vi "G2CPU GEMM And Operations Float.vi"(10 "Backend":T1 items=["Default Backend"=0, "CPU Backend"=1, "CUDA Backend"=2, "OPENCL Backend"=4, "Intel OneAPI"=8], 11 "dimension size":i32=16384) -> (3 "G2CPU Time":dbl)   [LabVIEW 2020]
uses:
  <vilib>/Natan Biesmans/G2CPU GPU and CPU HPC Toolkit/ArrayFire Driver/TypeDefs/backend.ctl
  ef11b89c-ff92-4b7a-88d6-625fca8c0d7c.vi
  c2200195-6f6b-46fb-afe8-d4cd0bcb91cf.vi
  fbbaf97c-3b5e-4b4c-bc14-40c3526c788b.vi
  ef11b89c-ff92-4b7a-88d6-625fca8c0d7c.vi/caaf1833-0905-411b-a9ed-2cc30d41907c.vi
  <vilib>/Natan Biesmans/G2CPU GPU and CPU HPC Toolkit/G2CPU Libraries/Arrays/SubVI/Array Sizes to Dim Cluster.vi
  c2200195-6f6b-46fb-afe8-d4cd0bcb91cf.vi/caaf1833-0905-411b-a9ed-2cc30d41907c.vi
  fbbaf97c-3b5e-4b4c-bc14-40c3526c788b.vi/caaf1833-0905-411b-a9ed-2cc30d41907c.vi
  ef11b89c-ff92-4b7a-88d6-625fca8c0d7c.vi/caaf1833-0905-411b-a9ed-2cc30d41907c.vi/c4afee3a-d58b-473f-ba2d-ee94fd2b49f4.vi
  c2200195-6f6b-46fb-afe8-d4cd0bcb91cf.vi/caaf1833-0905-411b-a9ed-2cc30d41907c.vi/c4afee3a-d58b-473f-ba2d-ee94fd2b49f4.vi
  fbbaf97c-3b5e-4b4c-bc14-40c3526c788b.vi/caaf1833-0905-411b-a9ed-2cc30d41907c.vi/c4afee3a-d58b-473f-ba2d-ee94fd2b49f4.vi
  <vilib>/Natan Biesmans/G2CPU GPU and CPU HPC Toolkit/G2CPU Libraries/Arrays/2DArray/f32/2D Array f32.lvclass
  C:/Program Files/National Instruments/LabVIEW 2020/vi.lib/Natan Biesmans/G2CPU GPU and CPU HPC Toolkit/G2CPU Libraries/Arrays/Array/Array Prototype.lvclass
  <vilib>/Natan Biesmans/G2CPU GPU and CPU HPC Toolkit/G2CPU Libraries/Runtime Licensing/G2CPU License Check.vi
  <vilib>/Natan Biesmans/G2CPU GPU and CPU HPC Toolkit/ArrayFire Driver/VIs/Run as Multi Device.vi
  <vilib>/Natan Biesmans/G2CPU GPU and CPU HPC Toolkit/G2CPU Libraries/Manage Environment/Find AF DLL.vi
  <vilib>/Natan Biesmans/G2CPU GPU and CPU HPC Toolkit/ArrayFire Driver/subvi/Error Converter (ErrCode or Status).vi
  <vilib>/Natan Biesmans/G2CPU GPU and CPU HPC Toolkit/G2CPU Libraries/Arrays/Array/G2CPU Set Array Pointer.vi
  <vilib>/Natan Biesmans/G2CPU GPU and CPU HPC Toolkit/G2CPU Libraries/Arrays/Array/Array Prototype.lvclass
  <vilib>/Natan Biesmans/G2CPU GPU and CPU HPC Toolkit/G2CPU Libraries/Manage Environment/G2CPU Manage Environment.lvlib
  <vilib>/Analysis/NI_AALBase.lvlib
  <vilib>/Natan Biesmans/G2CPU GPU and CPU HPC Toolkit/ArrayFire Driver/AF.lvlib
panel:
  out "max value":dbl
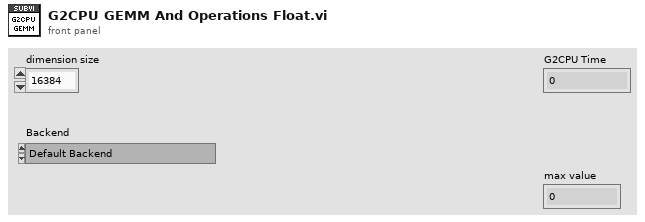
[diagram p1: front panel]
types:
  T1 = typedef "AF.lvlib/backend.ctl" = u32
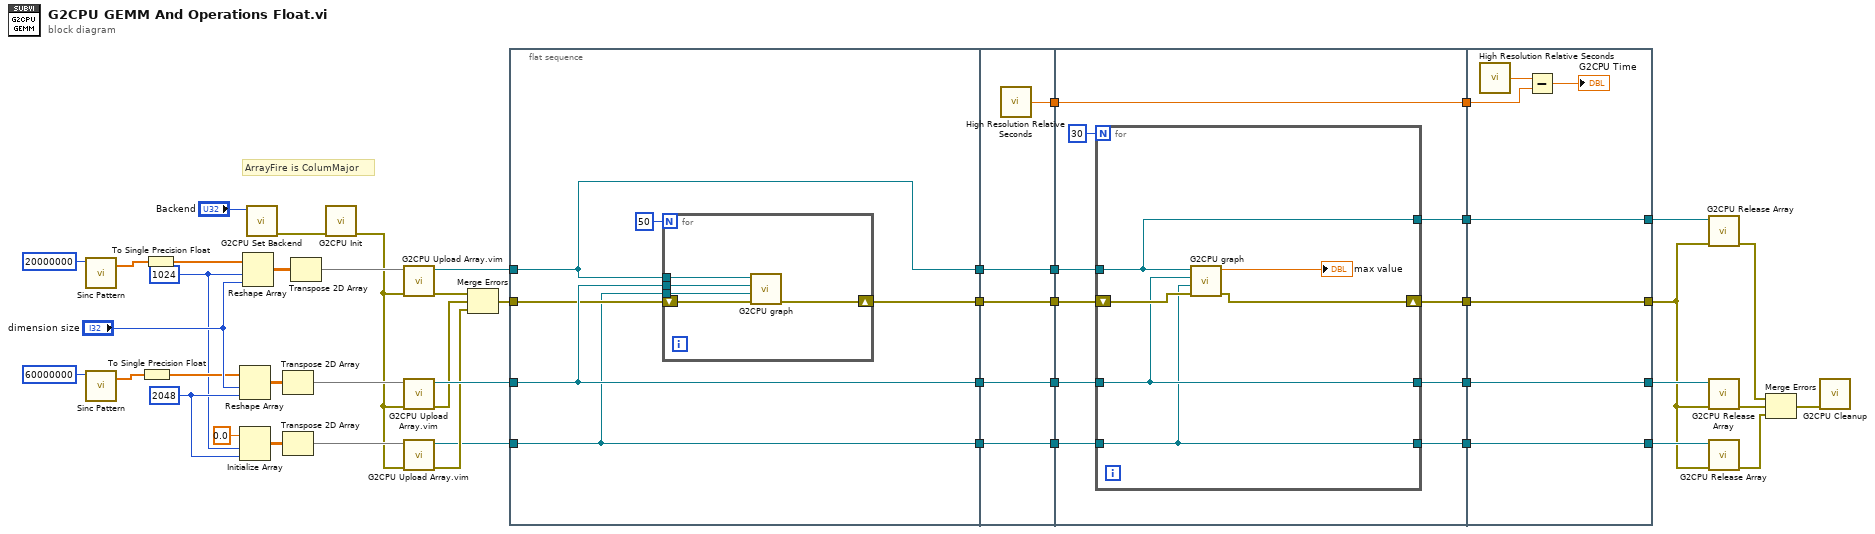
[diagram p0: block diagram]
diagram:
  w12 = 2048 ("dimension size")
  w11 = 1024 ("dimension size")
  # "ArrayFire is ColumMajor"
  n1 = call <vilib>:"Sinc Pattern.vi"("samples"=20000000) -> ("Sinc Pattern"=w43:dbl[])  [unwired: 3 in, 1 out]
  n2 = call <vilib>:"Sinc Pattern.vi"("samples"=60000000) -> ("Sinc Pattern"=w42:dbl[])  [unwired: 3 in, 1 out]
  n3 = To Single Precision Float(number=w42) -> (single precision float=w39:sgl[])
  n4 = To Single Precision Float(number=w43) -> (single precision float=w40:sgl[])
  n5 = Reshape Array(w39, "dimension size", w12) -> (w36:sgl[][])
  n6 = Initialize Array(sgl 0.0 ("element"), w11, w12) -> (w18:sgl[][])
  n7 = Reshape Array(w40, w11, "dimension size") -> (w35:sgl[][])
  n8 = call <vilib>:"G2CPU Set Backend.vi"("Backend"="Backend") -> ("error out"=w6:errorcluster)  [unwired: 10 in]
  n9 = Transpose 2D Array(2D array=w36) -> (transposed array=w22:sgl[][])
  n10 = Transpose 2D Array(2D array=w18) -> (transposed array=w19:sgl[][])
  n11 = Transpose 2D Array(2D array=w35) -> (transposed array=w23:sgl[][])
  n12 = call <vilib>:"G2CPU Init.vi"("error in (no error)"=w6) -> ("error out"=w5:errorcluster)  [unwired: 10 in]
  n13 = call "G2CPU Upload Array.vim"("error in (no error)"=w5, "Data"=w23) -> ("error out"=w30:errorcluster, "Array"=w34:refnum<class "2D Array f32.lvclass">)  [unwired: 8 in]
  n14 = call "G2CPU Upload Array.vim"("error in (no error)"=w5, "Data"=w22) -> ("error out"=w20:errorcluster, "Array"=w33:refnum<class "2D Array f32.lvclass">)  [unwired: 8 in]
  n15 = call "G2CPU Upload Array.vim"("error in (no error)"=w5, "Data"=w19) -> ("error out"=w17:errorcluster, "Array"=w16:refnum<class "2D Array f32.lvclass">)  [unwired: 8 in]
  n16 = Merge Errors(w30, w20, w17) -> (w21:errorcluster)
  n17 = flat-sequence {
    tunnel: w34 -> [w49]
    tunnel: [w49] -> w38
    tunnel: w33 -> [w53]
    tunnel: [w53] -> w32
    tunnel: w21 -> [w52]
    tunnel: [w54] -> w28
    tunnel: w16 -> [w51]
    tunnel: [w51] -> w14
    tunnel: [w64] -> w48
    tunnel: [w63] -> w47
    tunnel: w38 -> [w63]
    tunnel: w32 -> [w62]
    tunnel: [w62] -> w31
    tunnel: [w61] -> w29
    tunnel: w28 -> [w61]
    tunnel: [w60] -> w15
    tunnel: w14 -> [w60]
    tunnel: w48 -> [w74]
    tunnel: [w74] -> w46
    tunnel: w47 -> [w73]
    tunnel: [w71] -> w37
    tunnel: w31 -> [w70]
    tunnel: w29 -> [w69]
    tunnel: [w68] -> w25
    tunnel: w15 -> [w67]
    tunnel: [w66] -> w10
    tunnel: [w65] -> w9
    tunnel: w46 -> [w86]
    tunnel: w37 -> [w84]
    tunnel: [w84] -> w27
    tunnel: [w83] -> w26
    tunnel: w25 -> [w83]
    tunnel: [w82] -> w7
    tunnel: w10 -> [w82]
    tunnel: w9 -> [w81]
    tunnel: [w81] -> w8
    frame #0 {
      n18 = for {
        N: 50 -> [_]
        tunnel: w49 -> [w58]
        tunnel: w53 -> [w57]
        tunnel: w51 -> [w55]
        shift-right: [w59] -> w54
        shift-left: w52 -> [w56]
        n19 = call "G2CPU graph.vi"("error in (no error)"=w56, "C"=w55, "B"=w57, "A"=w58) -> ("error out"=w59:errorcluster)  [unwired: 6 in, 1 out]
      }
    }
    frame #1 {
      n20 = call <vilib>:"High Resolution Relative Seconds.vi"() -> ("relative seconds"=w64:dbl)
    }
    frame #2 {
      n21 = for {
        N: 30 -> [_]
        tunnel: w73 -> [w79]
        tunnel: [w79] -> w71
        tunnel: w70 -> [w78]
        tunnel: [w78] -> w68
        shift-right: [w76] -> w66
        shift-left: w69 -> [w80]
        tunnel: w67 -> [w75]
        tunnel: [w75] -> w65
        n22 = call "G2CPU graph.vi"("error in (no error)"=w80, "C"=w75, "B"=w78, "A"=w79) -> ("error out"=w76:errorcluster, "real out"=→"max value":dbl)  [unwired: 6 in]
      }
    }
    frame #3 {
      n23 = call <vilib>:"High Resolution Relative Seconds.vi"() -> ("relative seconds"=w87:dbl)
      n24 = Subtract(x=w87, y=w86) -> (x-y=→"G2CPU Time":dbl)
    }
  }
  n25 = call <vilib>:"G2CPU Release Array.vi"("error in (no error)"=w7, "Array in"=w27) -> ("error out"=w4:errorcluster)  [unwired: 9 in]
  n26 = call <vilib>:"G2CPU Release Array.vi"("error in (no error)"=w7, "Array in"=w26) -> ("error out"=w1:errorcluster)  [unwired: 9 in]
  n27 = call <vilib>:"G2CPU Release Array.vi"("error in (no error)"=w7, "Array in"=w8) -> ("error out"=w2:errorcluster)  [unwired: 9 in]
  n28 = Merge Errors(w4, w1, w2) -> (w3:errorcluster)
  n29 = call <vilib>:"G2CPU Cleanup.vi"("error in (no error)"=w3) -> ()  [unwired: 10 in, 1 out]
